vi "dont recreate channels test.vi"() -> ()   [LabVIEW 2014, in "Simple Sequencer TBM tests.lvlib"]
uses:
  <vilib>/NI/TBM Modules/Sequencer/testing/Simple Sequencer TBM tests.lvlib
  <vilib>/NI/TBM Modules/Sequencer/module/configuration/Simple Sequencer TBM configuration.lvclass
panel:
  out "created on first call":bool
  out "no subsequent creation":bool
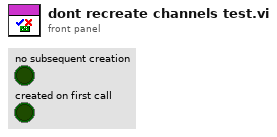
[diagram p1: front panel]
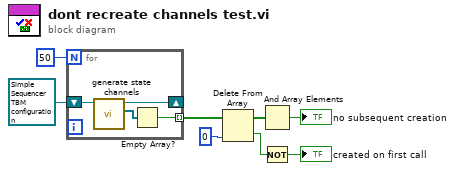
[diagram p0: block diagram]
diagram:
  n1 = for {
    N: 50 -> [_]
    tunnel: [w10] -> w8 mode=indexing
    shift-right: [w9] -> _
    shift-left: refnum<class "Simple Sequencer TBM configuration.lvclass"> refnum ("user module configuration") -> [w12]
    n2 = call <vilib>:"generate state channels.vi"("Simple Sequencer TBM configuration in"=w12) -> ("generated channels"=w11:refnum<class "TBM channel.lvclass">[], "Simple Sequencer TBM configuration out"=w9:refnum<class "Simple Sequencer TBM configuration.lvclass">)  [unwired: 9 in]
    n3 = Empty Array?(array=w11) -> (empty?=w10:bool)
  }
  n4 = Delete From Array(array=w8, index=0) -> (deleted portion=w4:bool, array with subset deleted=w6:bool[])  [unwired: 1 in]
  n5 = And Array Elements(Boolean array=w6) -> (logical AND=→"no subsequent creation":bool)
  n6 = Not(x=w4) -> (.not. x?=→"created on first call":bool)
